vi "mqtt register user events.vi"() -> (0 "Event Registration Refnum":refnum<event-registration>)   [LabVIEW 2017]
uses:
  mqtt-LabVIEW/src/class/mqtt/mqttTXqueue/mqttRXsubscriptionEventData.ctl
  mqtt-LabVIEW/src/class/mqtt/mqttTXqueue/mqttTXdataQueueFunction.ctl
  mqtt-LabVIEW/src/class/mqtt/mqttTXqueue/mqttRXsubscriptionEventFunction.ctl
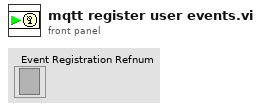
[diagram p1: front panel]
types:
  T1 = typedef "mqttRXsubscriptionEventFunction.ctl" = enum16{"init", "deinit", "getEventRef", "event"}
  T2 = typedef "mqttTXdataQueueFunction.ctl" = enum16{"init", "deinit", "getQueue", "enqueue"}
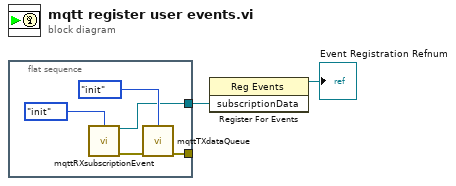
[diagram p0: block diagram]
diagram:
  n1 = flat-sequence {
    tunnel: [w6] -> _
    tunnel: [w3] -> w2
    frame #0 {
      n2 = call "mqttRXsubscriptionEvent.vi"("function"=mqttRXsubscriptionEventFunction."init") -> ("subscriptionData"=w3:refnum<user-event>, "error out"=w5:errorcluster)  [unwired: 13 in]
      n3 = call "mqttTXdataQueue.vi"("function"=mqttTXdataQueueFunction."init", "error in (no error)"=w5) -> ("error out"=w6:errorcluster)  [unwired: 12 in, 1 out]
    }
  }
  n4 = register-events(w2) -> (reference out=→"Event Registration Refnum":refnum<event-registration>)  [unwired: 2 in, 1 out]
